vi "WLAN - niVST - RFSA - Init.vi"(11 "RFSA Handle In":string) -> (0 "error out":errorcluster, 1 "IQ Meas Ref":T1, 2 "Spectrum Meas Ref":T1, 3 "RFSA Handle Out":refnum<k15>)   [LabVIEW 2012]
uses:
  <vilib>/RF Toolkits/WLAN/analysis/controls/wlanv1 Analysis Refnum.ctl
  <vilib>/RF Toolkits/WLAN/analysis/controls/wlanA version control.ctl
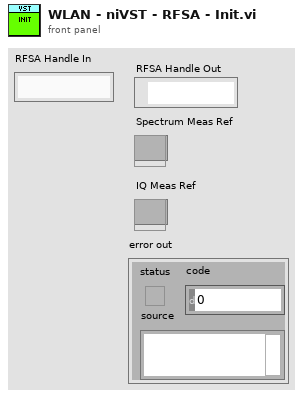
[diagram p1: front panel]
types:
  T1 = typedef "wlanv1 Analysis Refnum.ctl" = refnum<k20>
  T2 = typedef "wlanA version control.ctl" = i32
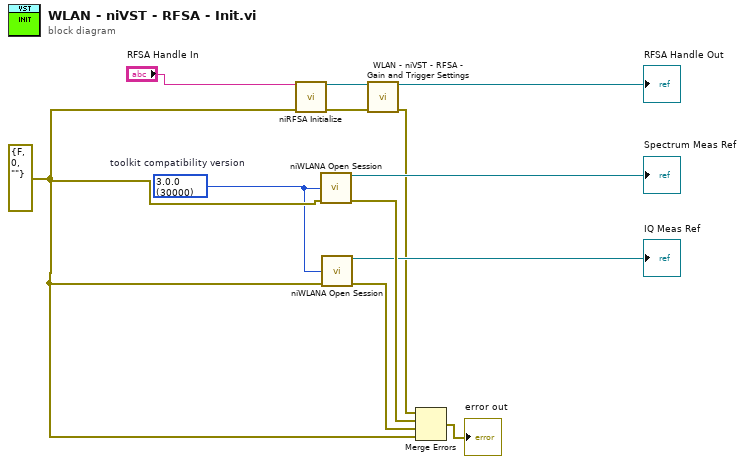
[diagram p0: block diagram]
diagram:
  w12 = errorcluster {"status"=FALSE, "code"=0, "source"=""} ("error in (no error)")
  w2 = T2 30000 items=["1.0.0"=10000, "2.0.0"=20000, "3.0.0"=30000]  # toolkit compatibility version
  n1 = call <instrlib>:"niRFSA Initialize.vi"("resource name"="RFSA Handle In", "error in"=w12) -> ("instrument handle"=w4:refnum<k15>, "error out"=w3:errorcluster)  [unwired: 12 in]
  n2 = call <vilib>:"niWLANA Open Session.vi"("toolkit compatibility version"=w2, "error in"=w12) -> ("niwlan analysis session"=→"Spectrum Meas Ref":T1, "error out"=w9:errorcluster)  [unwired: 11 in, 1 out]
  n3 = call <vilib>:"niWLANA Open Session.vi"("toolkit compatibility version"=w2, "error in"=w12) -> ("niwlan analysis session"=→"IQ Meas Ref":T1, "error out"=w7:errorcluster)  [unwired: 11 in, 1 out]
  n4 = call "WLAN - niVST - RFSA - Gain and Trigger Settings.vi"("instrument handle"=w4, "error in"=w3) -> ("instrument handle"=→"RFSA Handle Out":refnum<k15>, "error out"=w6:errorcluster)  [unwired: 12 in]
  n5 = Merge Errors(w6, w9, w7, w12) -> (→"error out":errorcluster)
